vi "Detection Logic to FPGA Modularized.vi"() -> ()   [LabVIEW 2026]
uses:
  <vilib>/rvi/Emulation/niFpgaGetClockAttributes.vi
  <vilib>/rvi/Emulation/niFpgaSctlEmulationGetInTimedLoop.vi
  <vilib>/rvi/Emulation/niFpgaEmulationReportErrorSimple.vi
  <extravilib>/ChannelInstances/Tag-u8/Instantiate.vi
  <extravilib>/ChannelInstances/Tag-bool/Instantiate.vi
  <vilib>/rvi/Emulation/niFpgaCriticalErrorInLSC.vi
  <vilib>/rvi/eio/common/nirviEmuTemplateMethod_errors.vi
  <vilib>/eio/EIONode/EIONode.xnode
  <extravilib>/ChannelInstances/Tag-bool.lvlib
  <extravilib>/ChannelInstances/Tag-u8.lvlib
panel:
  out "Score P2":u16
  out "Multiplier P2":u16
  out "Multiplier P1":u16
  out "Random Number":u8
  out "Score P1":u16
  in  "Speed Threshold, ticks":u64=3000
  in  "Debounce Threshold, ticks":u64=1000
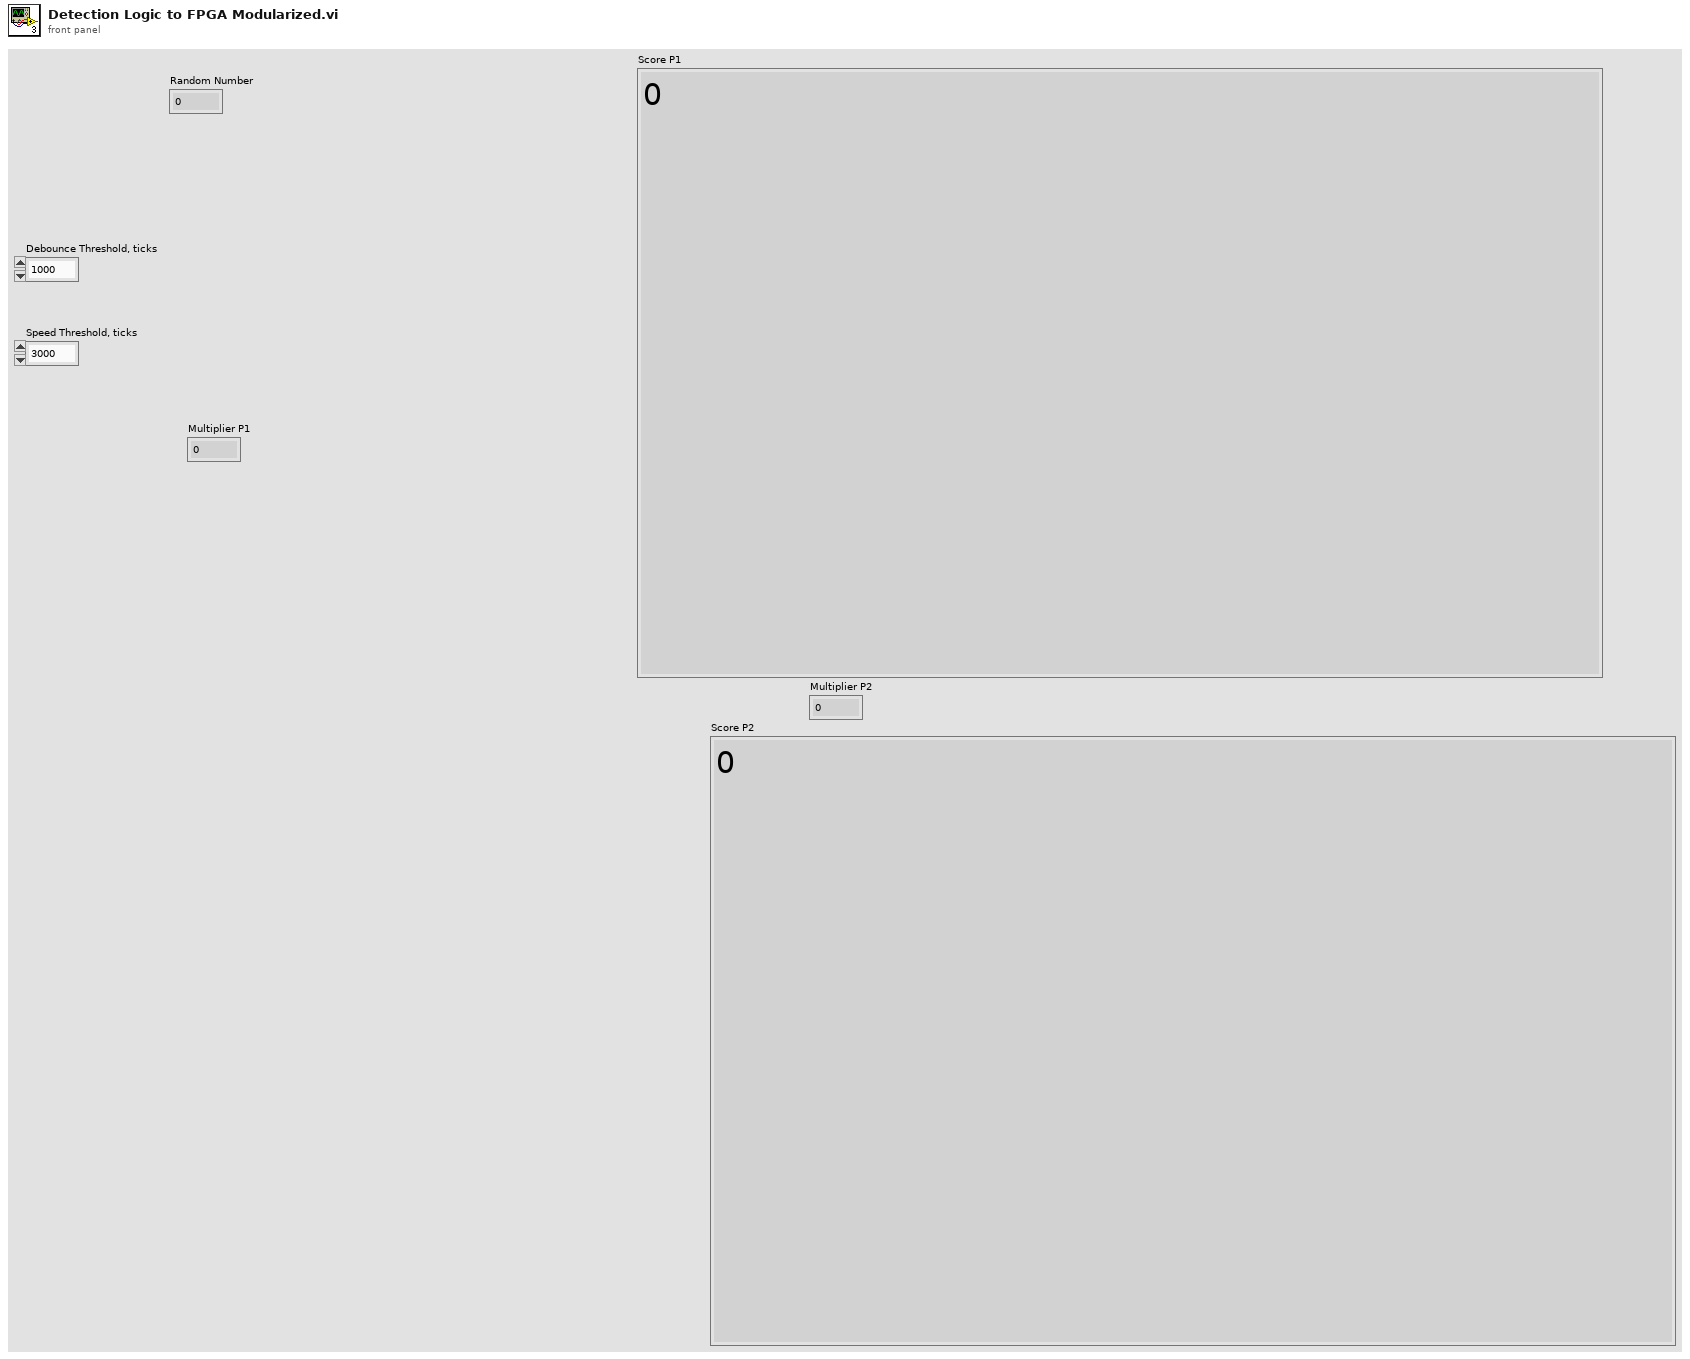
[diagram p1: front panel]
types:
  T1 = cluster{"Score":u16, "Multiplier":u16, "Last Press Tick":u64, u64[]}
  T2 = typedef "Tag-bool.lvlib/))Channel.ctl" = refnum<queue>
  T3 = cluster{"Score out":u16, "Multiplier out":u16, "Last Valid Press Tick out":u64, "Debounce Tick out":u64[]}
  T4 = typedef "Tag-u8.lvlib/))Channel.ctl" = refnum<queue>
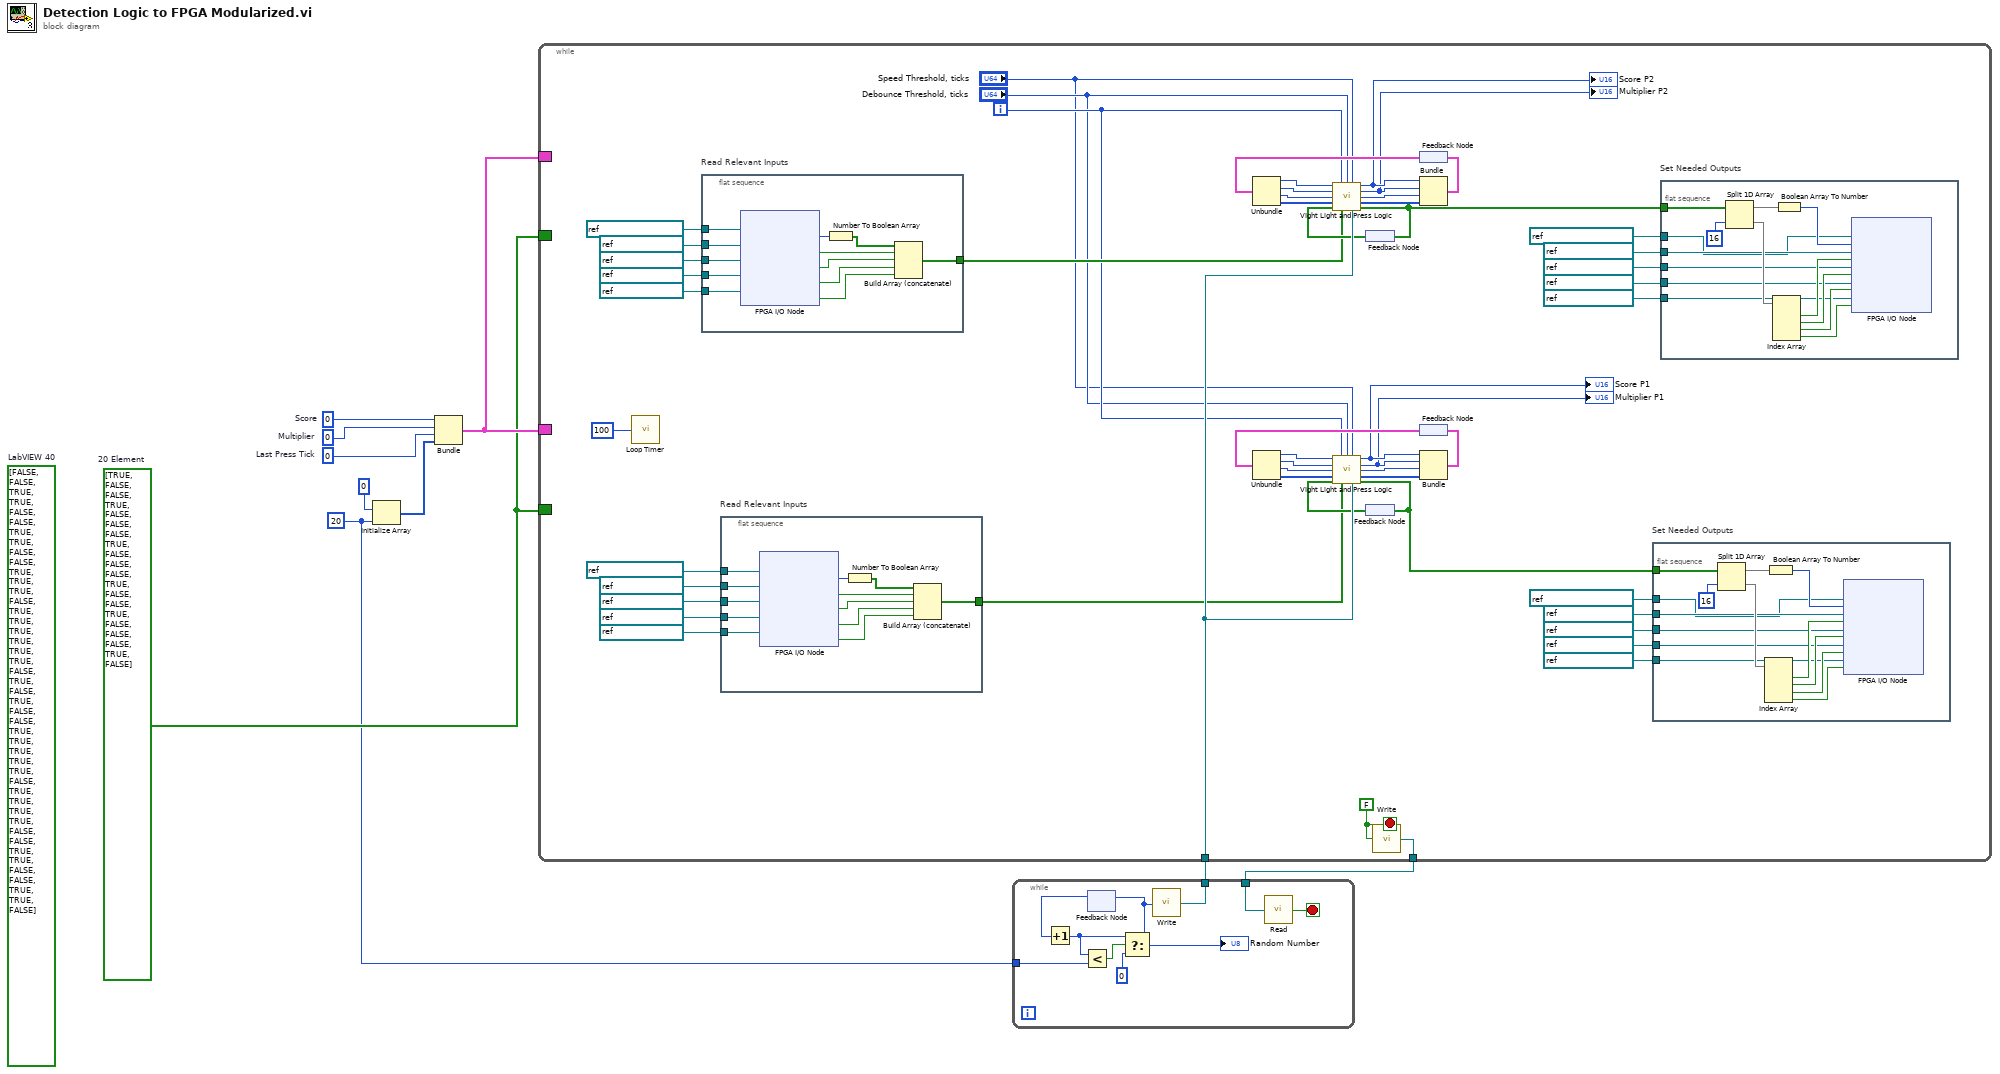
[diagram p0: block diagram]
diagram:
  (unwired) bool[] [FALSE, FALSE, TRUE, TRUE, FALSE, FALSE, TRUE, TRUE, FALSE, FALSE, TRUE, TRUE, TRUE, FALSE, TRUE, TRUE, TRUE, TRUE, TRUE, TRUE, FALSE, TRUE, FALSE, TRUE, FALSE, FALSE, TRUE, TRUE, TRUE, TRUE, TRUE, FALSE, TRUE, TRUE, TRUE, TRUE, FALSE, FALSE, TRUE, TRUE, FALSE, FALSE, TRUE, TRUE, FALSE]  # LabVIEW 40
  w6 = u64 0  # Last Press Tick
  w2 = 20 ("index")
  w3 = bool[] [TRUE, FALSE, FALSE, TRUE, FALSE, FALSE, FALSE, TRUE, FALSE, FALSE, FALSE, TRUE, FALSE, FALSE, TRUE, FALSE, FALSE, FALSE, TRUE, FALSE]  # 20 Element
  w7 = u16 0  # Multiplier
  w8 = u16 0  # Score
  n1 = Initialize Array(u64 0 ("Bonus Threshold"), w2) -> (w5:u64[])
  n2 = Bundle("Score"=w8, "Multiplier"=w7, "Last Press Tick"=w6, w5) -> (w4:T1)  [unwired: 1 in]
  n3 = while {
    tunnel: [w62] -> w1
    border: w3 -> [_]
    tunnel: w9 -> [w63]
    border: w4 -> [_]
    border: w3 -> [_]
    border: w4 -> [_]
    i -> [w13]
    stop <- w61 stop-if-true
    w61 = FALSE
    n4 = call "Loop Timer"("Count(uSec)"=u32 100) -> ()  [unwired: 1 out]
    n5 = flat-sequence "Read Relevant Inputs" {
      tunnel: [w78] -> w25
      tunnel: refnum<k21> "Bank-03/DI7" ("FPGA I/O In") -> [w83]
      tunnel: refnum<k21> "Bank-03/DI6" ("FPGA I/O In") -> [w82]
      tunnel: refnum<k21> "Bank-03/DI5" ("FPGA I/O In") -> [w81]
      tunnel: refnum<k21> "Bank-03/DI4" ("FPGA I/O In") -> [w80]
      tunnel: refnum<k21> "Bank-02/DI15:0" ("FPGA I/O In") -> [w79]
      frame #0 {
        n6 = xnode "FPGA I/O Node"("FPGA I/O In"=w79, "FPGA I/O In"=w80, "FPGA I/O In"=w81, "FPGA I/O In"=w82, "FPGA I/O In"=w83) -> ("I/O Item"=w84:u16, "I/O Item"=w86:bool, "I/O Item"=w87:bool, "I/O Item"=w88:bool, "I/O Item"=w89:bool)  [unwired: 5 out]
        n7 = Number To Boolean Array(number=w84) -> (Boolean array=w85:bool[])
        n8 = Build Array (concatenate)(w85, w86, w87, w88, w89) -> (w78:bool[])
      }
    }
    n9 = flat-sequence "Read Relevant Inputs" {
      tunnel: [w109] -> w47
      tunnel: refnum<k21> "Bank-03/DI3" ("FPGA I/O In") -> [w108]
      tunnel: refnum<k21> "Bank-03/DI2" ("FPGA I/O In") -> [w107]
      tunnel: refnum<k21> "Bank-03/DI1" ("FPGA I/O In") -> [w106]
      tunnel: refnum<k21> "Bank-03/DI0" ("FPGA I/O In") -> [w105]
      tunnel: refnum<k21> "Bank-01/DI15:0" ("FPGA I/O In") -> [w104]
      frame #0 {
        n10 = xnode "FPGA I/O Node"("FPGA I/O In"=w104, "FPGA I/O In"=w105, "FPGA I/O In"=w106, "FPGA I/O In"=w107, "FPGA I/O In"=w108) -> ("I/O Item"=w110:u16, "I/O Item"=w112:bool, "I/O Item"=w113:bool, "I/O Item"=w114:bool, "I/O Item"=w115:bool)  [unwired: 5 out]
        n11 = Number To Boolean Array(number=w110) -> (Boolean array=w111:bool[])
        n12 = Build Array (concatenate)(w111, w112, w113, w114, w115) -> (w109:bool[])
      }
    }
    n13 = feedback #1() -> (w38:bool[])
    n14 = feedback #2() -> (w59:bool[])
    n15 = call <extravilib>:"Write.vi"("element"=w61) -> ("channel"=w62:T2)  [unwired: 1 out]
    n16 = feedback #3() -> (w42:T1)
    n17 = Unbundle(w42) -> ("Score"=w43:u16, "Multiplier"=w44:u16, "Last Press Tick"=w45:u64, w46:u64[])
    n18 = call "VIght Light and Press Logic.vi"("Score in"=w43, "Tick"=w13, "Debounce Threshold, ticks"="Debounce Threshold, ticks", "Speed Threshold, ticks"="Speed Threshold, ticks", "Multiplier in"=w44, "Last Valid Press Tick in"=w45, "Debounce Tick in"=w46, "Lit Buttons"=w38, "Pressed Buttons"=w25, "Random Number"=w63) -> ("Score out"=w37:u16, "Multiplier out"=w36:u16, "Last Valid Press Tick out"=w40:u64, "Debounce Tick out"=w39:u64[], "Buttons to Light"=w19:bool[])  [unwired: 1 in]
    "Score P2" <- w37
    "Multiplier P2" <- w36
    n19 = feedback-in #1(w19) -> ()
    n20 = Bundle("Score out"=w37, "Multiplier out"=w36, "Last Valid Press Tick out"=w40, "Debounce Tick out"=w39) -> (w41:T3)  [unwired: 1 in]
    n21 = feedback-in #3(w41) -> ()
    n22 = feedback #4() -> (w54:T1)
    n23 = Unbundle(w54) -> ("Score"=w53:u16, "Multiplier"=w52:u16, "Last Press Tick"=w51:u64, w50:u64[])
    n24 = call "VIght Light and Press Logic.vi"("Score in"=w53, "Tick"=w13, "Debounce Threshold, ticks"="Debounce Threshold, ticks", "Speed Threshold, ticks"="Speed Threshold, ticks", "Multiplier in"=w52, "Last Valid Press Tick in"=w51, "Debounce Tick in"=w50, "Lit Buttons"=w59, "Pressed Buttons"=w47, "Random Number"=w63) -> ("Score out"=w49:u16, "Multiplier out"=w48:u16, "Last Valid Press Tick out"=w56:u64, "Debounce Tick out"=w57:u64[], "Buttons to Light"=w58:bool[])  [unwired: 1 in]
    "Score P1" <- w49
    "Multiplier P1" <- w48
    n25 = feedback-in #2(w58) -> ()
    n26 = Bundle("Score out"=w49, "Multiplier out"=w48, "Last Valid Press Tick out"=w56, "Debounce Tick out"=w57) -> (w55:T3)  [unwired: 1 in]
    n27 = feedback-in #4(w55) -> ()
    n28 = flat-sequence "Set Needed Outputs" {
      tunnel: w58 -> [w103]
      tunnel: refnum<k21> "Bank-03/DO3" ("FPGA I/O In") -> [w90]
      tunnel: refnum<k21> "Bank-03/DO2" ("FPGA I/O In") -> [w94]
      tunnel: refnum<k21> "Bank-03/DO1" ("FPGA I/O In") -> [w93]
      tunnel: refnum<k21> "Bank-03/DO0" ("FPGA I/O In") -> [w92]
      tunnel: refnum<k21> "Bank-01/DO15:0" ("FPGA I/O In") -> [w91]
      frame #0 {
        n29 = Split 1D Array(array=w103, index=16) -> (first subarray=w101:bool[], second subarray=w99:bool[])
        n30 = Index Array(array=w99) -> (element #1=w98:bool, element #2=w97:bool, element #3=w96:bool, element #4=w95:bool)  [unwired: 4 in]
        n31 = Boolean Array To Number(Boolean array=w101) -> (number=w102:u16)
        n32 = xnode "FPGA I/O Node"("I/O Item"=w102, "FPGA I/O In"=w91, "I/O Item"=w98, "FPGA I/O In"=w92, "I/O Item"=w97, "FPGA I/O In"=w93, "I/O Item"=w96, "FPGA I/O In"=w94, "I/O Item"=w95, "FPGA I/O In"=w90) -> ()  [unwired: 5 out]
      }
    }
    n33 = flat-sequence "Set Needed Outputs" {
      tunnel: w19 -> [w77]
      tunnel: refnum<k21> "Bank-03/DO7" ("FPGA I/O In") -> [w64]
      tunnel: refnum<k21> "Bank-03/DO6" ("FPGA I/O In") -> [w68]
      tunnel: refnum<k21> "Bank-03/DO5" ("FPGA I/O In") -> [w67]
      tunnel: refnum<k21> "Bank-03/DO4" ("FPGA I/O In") -> [w66]
      tunnel: refnum<k21> "Bank-02/DO15:0" ("FPGA I/O In") -> [w65]
      frame #0 {
        n34 = Split 1D Array(array=w77, index=16) -> (first subarray=w75:bool[], second subarray=w73:bool[])
        n35 = Index Array(array=w73) -> (element #1=w72:bool, element #2=w71:bool, element #3=w70:bool, element #4=w69:bool)  [unwired: 4 in]
        n36 = Boolean Array To Number(Boolean array=w75) -> (number=w76:u16)
        n37 = xnode "FPGA I/O Node"("I/O Item"=w76, "FPGA I/O In"=w65, "I/O Item"=w72, "FPGA I/O In"=w66, "I/O Item"=w71, "FPGA I/O In"=w67, "I/O Item"=w70, "FPGA I/O In"=w68, "I/O Item"=w69, "FPGA I/O In"=w64) -> ()  [unwired: 5 out]
      }
    }
  }
  n38 = while {
    tunnel: w1 -> [w120]
    tunnel: w2 -> [w117]
    tunnel: [w116] -> w9
    stop <- w119 stop-if-true
    n39 = feedback #5() -> (w122:u8)  [unwired: 1 in]
    n40 = Increment(x=w122) -> (x+1=w118:u8)
    n41 = Less?(x=w118, y=w117) -> (x < y?=w123:bool)
    n42 = Select(t=w118, s=w123, f=u8 0) -> (s? t:f=w124:u8)
    "Random Number" <- w124
    n43 = feedback-in #5(w124) -> ()
    n44 = call <extravilib>:"Write.vi"("element"=w124) -> ("channel"=w116:T4)  [unwired: 1 out]
    n45 = call <extravilib>:"Read.vi"("channel"=w120) -> ("element"=w119:bool)  [unwired: 1 in, 1 out]
  }
